vi "X-Axis_Generator_f.vi"(0 "File Info In":T2={"FilePath"=path "/DATA/Labview Items", "Field (T)"=12.0, "Temperature (K)"=12.0, "X-Axis"=enum."nm", "Center nm"=-1.0, "Current Grating Density"=enum."600", "CCD Parameters"={"Exposure Time (s)"=0.2, "Offset"=0.0, "BkgrdCrct"=FALSE, "Shutter"=FALSE, "Mode"=enum."Regular", "Repetition"=4, "dt or s"=0.0}, "Operation Mode"=enum."NML Data Acquisition", "Exp Index"=3, "Index_repetition"=0, "Index"=0, "Current Detector"=enum."CCD-1024x256"} {"CCD Parameters"."dt or s" format="%#.6f"; "CCD Parameters"."Repetition" min=1; "CCD Parameters"."Offset" format="%#.2f"; "CCD Parameters"."Exposure Time (s)" min=0.02 max=6000.0 format="%#.2f"; "Center nm" format="%.2f"; "Temperature (K)" format="%.2f"; "Field (T)" format="%.2f"}, 2 "Current Grating Density":T4=enum."600" caption="Grating Density", 5 "X-Axis Unit":T3=enum."nm", 7 "Current Detector":T1, 8 "X-Axis Points":enum16{"1024", "512", "3"}(ring)) -> (12 "X-axis  (nm)":dbl[](array[numeric])=[571.2504622529284, 585.6489231225254, 600.0000000000001, 614.300024178551, 628.5453659653462] format="%.4f", 13 "X-axis":dbl[](array[numeric])=[571.2504622529284, 585.6489231225254, 600.0000000000001, 614.300024178551, 628.5453659653462] format="%.4f", 14 "nm (Max)":dbl=628.5453659653462 format="%.4f", 15 "nm (Min)":dbl=571.2504622529284 format="%.4f", 16 "cm-1 (Max)":dbl=17505.45629418217 format="%.2f", 17 "cm-1 (Min)":dbl=15909.750578848963 format="%.2f", 18 "meV (Max)":dbl=2170.4007572687524 format="%.2f", 19 "meV (Min)":dbl=1972.5583911666886 format="%.2f")   [LabVIEW 2020]
doc: "Generate CCD X-array.\nInput can be either from the fileInfo Cluster or from the individual components."
uses:
  Globals and TypeDefs/Type Definitions.llb/McPherson Grating Density.ctl
  Globals and TypeDefs/Type Definitions.llb/Wavelength Unit.ctt
  Globals and TypeDefs/Type Definitions.llb/FileInfoParameter.ctt
  Globals and TypeDefs/Type Definitions.llb/CCDParameter.ctt
  Globals and TypeDefs/Type Definitions.llb/OperationMode.ctt
  Globals and TypeDefs/Type Definitions.llb/ListOfDetectors.ctt
  X-Axis Converter.llb/X-Axis Converter.vi
panel:
  out "nm (delta)":dbl=57.29490371241775 format="%.4f"
  out "cm-1 (delta)":dbl=1595.705715333208 format="%.2f"
  out "meV (delta)":dbl=197.8423661020638 format="%.2f"
  out "Detector Pixel Distance":dbl=27.0 format="%.2f"
  out "beta":dbl=0.03851514953863218 format="%.2f"
  out "alpha":dbl=21.141484850461367 format="%.2f"
  out "Spectrometer Mirror angle":dbl=21.18 format="%.2f"
  out "Spectrometer Focal length":dbl=750.0 format="%.1f"
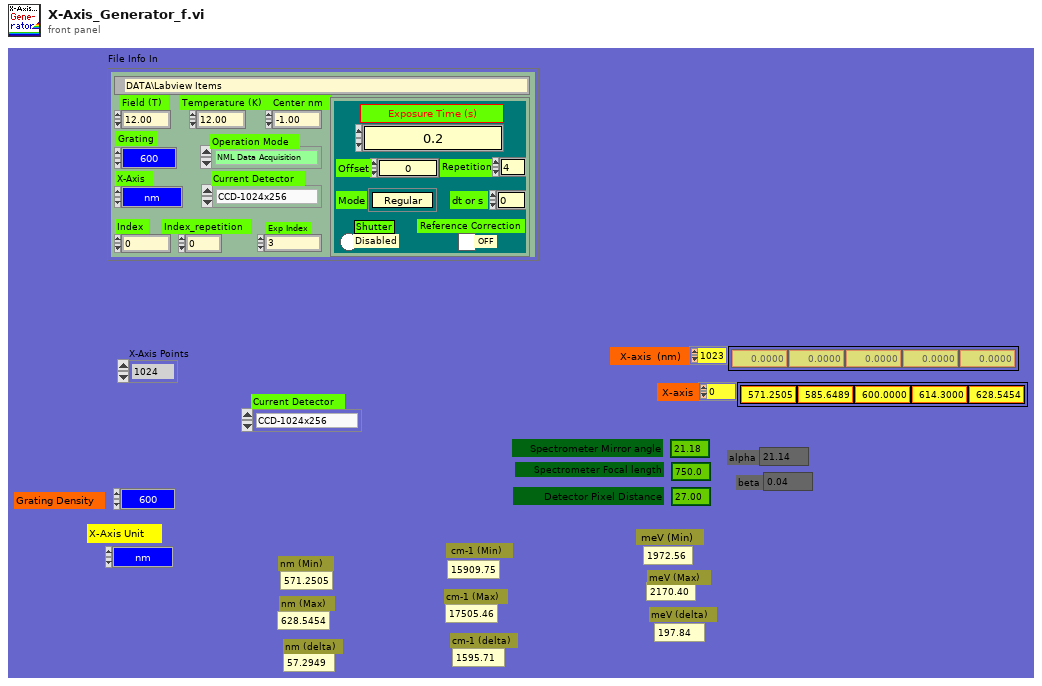
[diagram p1: front panel]
types:
  T1 = typedef "ListOfDetectors.ctt" = enum8{"CCD-1024x256", "InGaAs PDA-1024x1", "CCD-1340x400", "Ge Single Channel", "Si Single Channel", "PMT Single Channel"}
  T2 = typedef "FileInfoParameter.ctt" = cluster{"FilePath":path, "Field (T)":dbl, "Temperature (K)":dbl, "X-Axis":T3, "Center nm":dbl, "Current Grating Density":T4, "CCD Parameters":T5, "Operation Mode":T6, "Exp Index":u32, "Index_repetition":u16, "Index":u16, "Current Detector":T1}
  T3 = typedef "Wavelength Unit.ctt" = enum8{"Point", "nm", "eV", "meV", "cm_1"}
  T4 = typedef "McPherson Grating Density.ctl" = enum8{"150", "300", "600", "1200", "1800"}
  T5 = typedef "CCDParameter.ctt" = cluster{"Exposure Time (s)":dbl, "Offset":dbl, "BkgrdCrct":bool, "Shutter":bool, "Mode":enum8{"Regular", "OverExp Cor", "SpikeRemove", "ForCalibration"}, "Repetition":u16, "dt or s":dbl}
  T6 = typedef "OperationMode.ctt" = enum16{"Standby", "CCD Single Shot", "CCD Sequence Shots", "CCD Custom Shots", "CCD Reference Shot", "Step Scanning ", "Time Scanning", "NML Data Acquisition"}
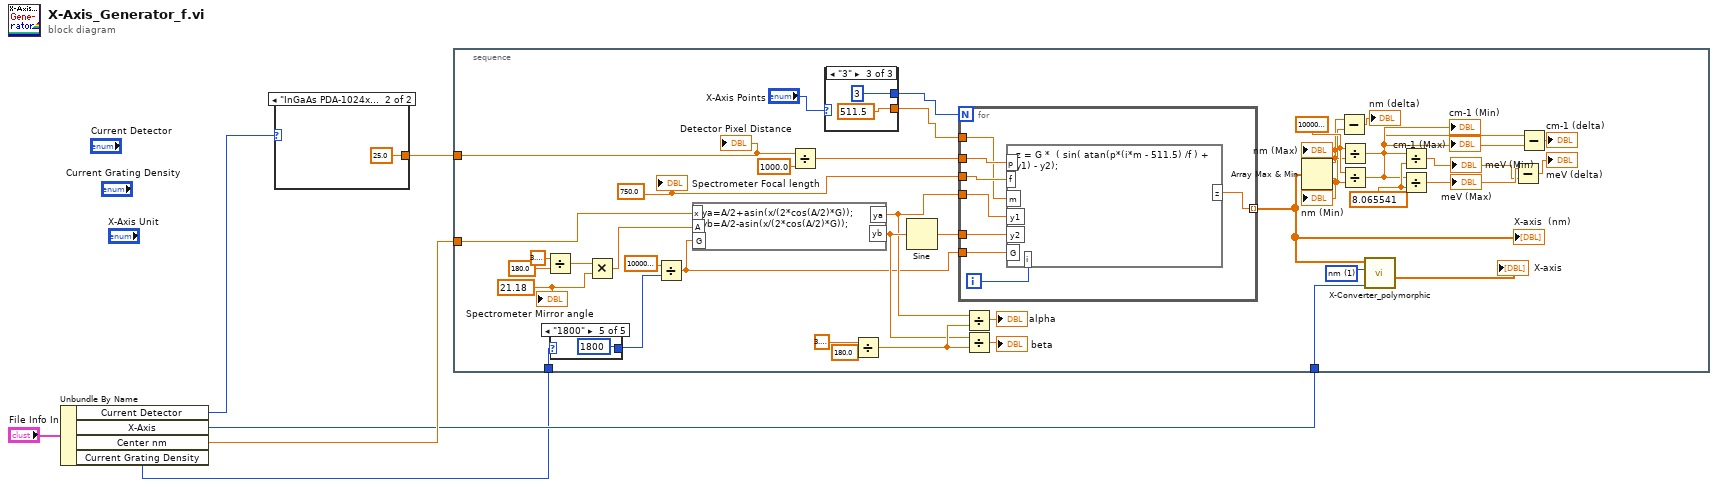
[diagram p0: block diagram]
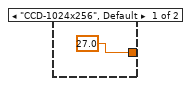
[diagram p2: hidden frame]
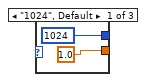
[diagram p3: hidden frame]
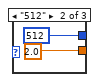
[diagram p4: hidden frame]
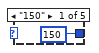
[diagram p5: hidden frame]
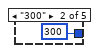
[diagram p6: hidden frame]
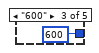
[diagram p7: hidden frame]
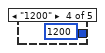
[diagram p8: hidden frame]
diagram:
  n1 = Unbundle By Name("File Info In") -> ("Current Detector"=w2:T1, "X-Axis"=w4:T3, "Center nm"=w5:dbl, "Current Grating Density"=w3:T4)
  n2 = case shown="\"InGaAs PDA-1024x1\"" w2 {
    tunnel: [27.0 ("x") 25.0 ("x")] -> w1
    frame "CCD-1024x256", Default {
    }
    frame "InGaAs PDA-1024x1" {
    }
  }
  n3 = stacked-sequence {
    tunnel: w3 -> [w21]
    tunnel: w5 -> [w20]
    tunnel: w4 -> [w19]
    tunnel: w1 -> [w9]
    frame #0 {
      w23 = 1 items=["Point #", "nm", "eV", "meV", "cm-1"] ("Old X-Axis Unit")
      w33 = 21.18 ("Detector Pixel Distance")
      w14 = 750.0 ("Detector Pixel Distance")
      w43 = 8.065541
      w44 = 10000000.0
      n4 = Divide(x=3.141592653589793, y=180.0) -> (x/y=w28:dbl)
      n5 = case shown="\"1800\"" w21 {
        tunnel: [150 300 600 1200 1800] -> w25
        frame "150" {
        }
        frame "300" {
        }
        frame "600" {
        }
        frame "1200" {
        }
        frame "1800" {
        }
      }
      n6 = Multiply(x=w28, y=w33) -> (x*y=w32:dbl)
      n7 = Divide(x=1000000.0, y=w25) -> (x/y=w11:dbl)
      n8 = formula code="ya=A/2+asin(x/(2*cos(A/2)*G));\nyb=A/2-asin(x/(2*cos(A/2)*G));"("x"=w20, "A"=w32, "G"=w11) -> ("ya"=w13:dbl, "yb"=w26:dbl)
      n9 = Divide(x=w9, y=1000.0) -> (x/y=w15:dbl)
      n10 = case shown="\"3\"" "X-Axis Points" {
        tunnel: [1024 512 3] -> w17
        tunnel: [1.0 2.0 511.5] -> w16
        frame "1024", Default {
        }
        frame "512" {
        }
        frame "3" {
        }
      }
      n11 = Divide(x=3.141592653589793, y=180.0) -> (x/y=w31:dbl)
      n12 = Sine(x=w26) -> (sin(x)=w10:dbl)
      n13 = for {
        N: w17 -> [_]
        tunnel: w15 -> [w55]
        tunnel: w14 -> [w54]
        tunnel: w16 -> [w53]
        tunnel: w13 -> [w52]
        tunnel: w10 -> [w51]
        tunnel: w11 -> [w50]
        tunnel: [w49] -> w12 mode=indexing
        i -> [w56]
        n14 = formula code="z = G *  ( sin( atan(p*(i*m - 511.5) /f ) + y1) - y2);"("p"=w55, "f"=w54, "m"=w53, "y1"=w52, "y2"=w51, "G"=w50, "i"=w56) -> ("z"=w49:dbl)
      }
      "X-axis  (nm)" <- w12
      n15 = Divide(x=w13, y=w31) -> (x/y=→"alpha":dbl)
      n16 = Divide(x=w26, y=w31) -> (x/y=→"beta":dbl)
      n17 = Array Max & Min(array=w12) -> (max value=w37:dbl, min value=w36:dbl)  [unwired: 2 out]
      "nm (Max)" <- w37
      "nm (Min)" <- w36
      n18 = Subtract(x=w37, y=w36) -> (x-y=→"nm (delta)":dbl)
      n19 = Divide(x=w44, y=w37) -> (x/y=w41:dbl)
      "cm-1 (Min)" <- w41
      n20 = Divide(x=w44, y=w36) -> (x/y=w40:dbl)
      "cm-1 (Max)" <- w40
      n21 = call-poly "X-Converter_polymorphic.vi"("X-Axis Unit"=w19, "Old X-Axis Unit"=w23, "X-Axis input"=w12) -> ("X-Axis Output"=→"X-axis":dbl[])  [unwired: 2 in, 3 out]
      n22 = Divide(x=w41, y=w43) -> (x/y=w39:dbl)
      "meV (Min)" <- w39
      n23 = Divide(x=w40, y=w43) -> (x/y=w42:dbl)
      "meV (Max)" <- w42
      n24 = Subtract(x=w42, y=w39) -> (x-y=→"meV (delta)":dbl)
      n25 = Subtract(x=w40, y=w41) -> (x-y=→"cm-1 (delta)":dbl)
      "Spectrometer Focal length" <- w14
      "Spectrometer Mirror angle" <- w33
      "Detector Pixel Distance" <- w9
    }
  }
